vi "题目4.1.vi"() -> ()   [LabVIEW 2017]
panel:
  in  "枚举":enum16{"张三", "李四", "王五"}(ring)
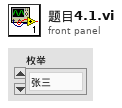
[diagram p1: front panel]
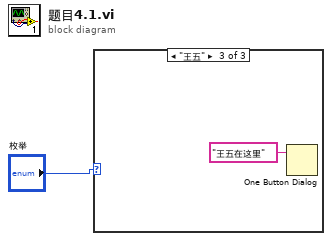
[diagram p0: block diagram]
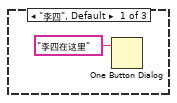
[diagram p2: hidden frame]
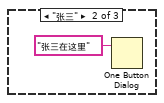
[diagram p3: hidden frame]
diagram:
  n1 = case shown="\"王五\"" "枚举" {
    frame "李四", Default {
      n2 = One Button Dialog(message="李四在这里" ("消息")) -> ()  [unwired: 1 in, 1 out]
    }
    frame "张三" {
      n3 = One Button Dialog(message="张三在这里" ("消息")) -> ()  [unwired: 1 in, 1 out]
    }
    frame "王五" {
      n4 = One Button Dialog(message="王五在这里" ("消息")) -> ()  [unwired: 1 in, 1 out]
    }
  }
